vi "HMI.vi"(8 "error in (no error)":errorcluster caption="entrée d'erreur (pas d'erreur)", 11 "Class Popup WaitDIO en entrée":refnum<class "Class Popup WaitDIO.lvclass">) -> (0 "error out":errorcluster caption="sortie d'erreur", 1 "Input":string, 2 "Operator_Selection":bool, 3 "Class Popup WaitDIO en sortie":refnum<class "Class Popup WaitDIO.lvclass">)   [LabVIEW 2020, in "Library Instrument & Equipement.lvlib" / "Library Popup.lvlib" / "Class Popup WaitDIO.lvclass"]
uses:
  Class Popup WaitDIO.lvclass
  C:/Users/ngarcin/OneDrive - Altyor/Standard TB/Class/Popup/Class Popup (Main)/Class Popup (Main).lvclass
  C:/Users/ngarcin/OneDrive - Altyor/Standard TB/Class/Popup/Class Popup Operator_Validation/Class Popup Operator_Validation (Default)/Class Popup Operator_Validation (Virtual).lvclass
  Commun VI/TypeDef/Liste Error.ctl
  JSON API/JSON Value/Set from JSON string.vi
  Instrument/Instrument (Default)/Class Instrument (Default).lvclass
  JSON API/JSON Value/JSON Value.lvclass
  Class Popup Operator_Validation/Class Popup Operator_Validation (Default)/Class Popup Operator_Validation (Virtual).lvclass
  Class Popup WaitDIO.lvclass/Class Popup WaitDIO.ctl
  JSON API/Variant JSON/Variant JSON.lvlib
  JSON API/Get Polymorphic/JSON GetSet.lvlib
  Commun VI/Library Commun.lvlib
panel:
  out "Json_String":string
  out "Image":picture
  out "Text":string
  in  "Bouton NOK":bool caption="Default"
  in  "Bouton OK":bool caption="Validated"
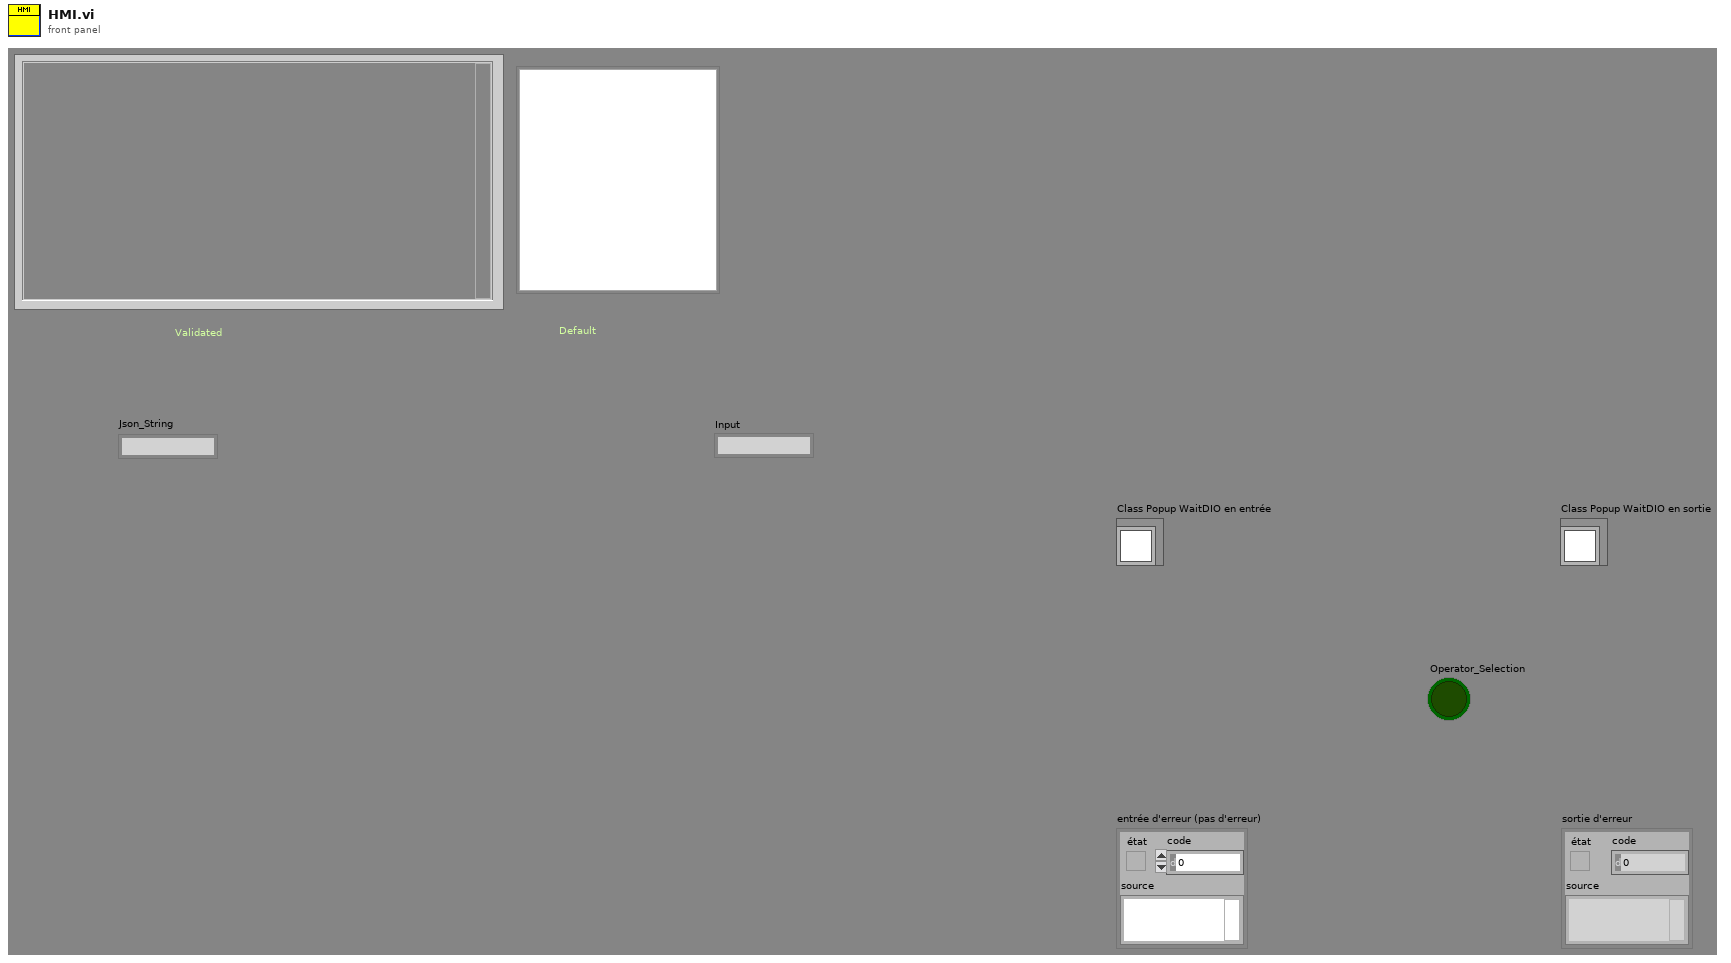
[diagram p1: front panel]
types:
  T1 = cluster{"Instrument":refnum<class "Class Instrument (Default).lvclass">, "Valur for test":bool, "Timeout (ms)":u64}
  T2 = typedef "Library Commun.lvlib/Liste Error.ctl" = enum16{"Firebase Driver - Get Document", "Firebase Driver - Get Document With Where", "Firebase Driver - Delete Document", "Firebase Driver - Set Document", "Firebase Driver - Update Document", "Firebase Altyor - Search Document Bench", "Firebase Altyor - Class Not in Firebase", "Spectrum_Analyser - Timeout", "Relay Board - Qty Relay", "DIO - Pb Funtion", "Power_Supply - Peripherical not find", "Mutimeter - Peripherical not find", "Instrument - Function Not Used", "Instrument - Instrument name not specified", "Instrument - Allready Initialised", "Instrument - TimeOut", "Instrument - the instrument must be Initialise before", "Instrument - Frame Not received", "Instrument - Frame Nok", "Test - Initialise the File_for_Save", "Test - Timeout", "Test - Cmd Error", "FGV - Variable ", "BDD FireBase - Define Class", "SN - Class Not Define"}
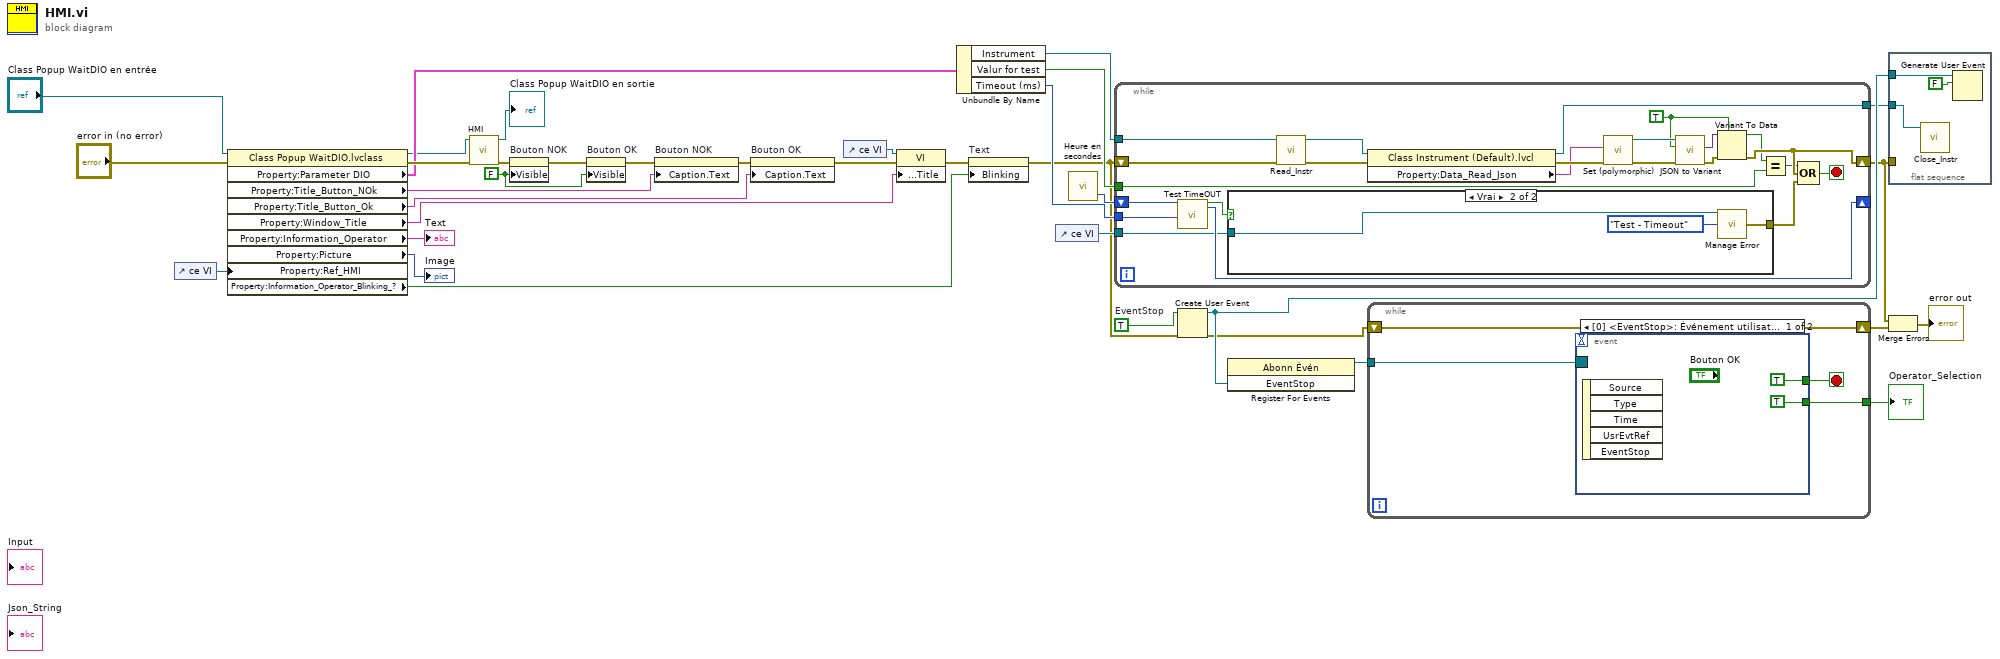
[diagram p0: block diagram]
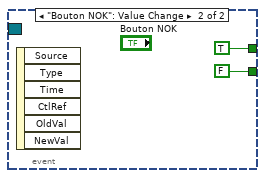
[diagram p3: hidden frame]
diagram:
  w18 = TRUE  # EventStop
  w22 = FALSE ("Visible")
  n1 = control-ref of="ce VI"() -> (w27:refnum<vi>)
  n2 = property class="Class Popup WaitDIO.lvclass"(reference="Class Popup WaitDIO en entrée", error in="error in (no error)", "Property:Ref_HMI"=w27) -> (reference out=w2:refnum<class "Class Popup WaitDIO.lvclass">, error out=w11:errorcluster, "Property:Parameter DIO"=w4:T1, "Property:Title_Button_NOk"=w35:string, "Property:Title_Button_Ok"=w36:string, "Property:Window_Title"=w30:string, "Property:Information_Operator"=→"Text":string, "Property:Picture"=→"Image":picture, "Property:Information_Operator_Blinking_?"=w25:bool)
  n3 = call-parent "HMI.vi"("error in (no error)"=w11, "Class Popup Operator_Validation (Default) en entrée"=w2) -> ("error out"=w3:errorcluster, "Class Popup Operator_Validation (Default) en sortie"=→"Class Popup WaitDIO en sortie":refnum<class "Class Popup WaitDIO.lvclass">)  [unwired: 6 in, 2 out]
  n4 = property on="Bouton NOK" class="Bool"(error in=w3, "Visible"=w22) -> (error out=w34:errorcluster)  [unwired: 1 in, 1 out]
  n5 = property on="Bouton OK" class="Bool"(error in=w34, "Visible"=w22) -> (error out=w33:errorcluster)  [unwired: 1 in, 1 out]
  n6 = property on="Bouton NOK" class="Bool"(error in=w33, "Caption.Text"=w35) -> (error out=w32:errorcluster)  [unwired: 1 in, 1 out]
  n7 = property on="Bouton OK" class="Bool"(error in=w32, "Caption.Text"=w36) -> (error out=w10:errorcluster)  [unwired: 1 in, 1 out]
  n8 = control-ref of="ce VI"() -> (w31:refnum<vi>)
  n9 = property class="VI"(reference=w31, error in=w10, "Front Panel.Title"=w30) -> (error out=w26:errorcluster)  [unwired: 1 out]
  n10 = Unbundle By Name(w4) -> ("Instrument"=w7:refnum<class "Class Instrument (Default).lvclass">, "Valur for test"=w12:bool, "Timeout (ms)"=w13:u64)
  n11 = property on="Text" class="Ch"(error in=w26, "Blinking"=w25) -> (error out=w6:errorcluster)  [unwired: 1 in, 1 out]
  n12 = control-ref of="ce VI"() -> (w20:refnum<vi>)
  n13 = call "Heure en secondes.vi"() -> ("Heure en milisecondes"=w21:u32)  [unwired: 2 in, 1 out]
  n14 = while {
    tunnel: w7 -> [w59]
    shift-right: [w48] -> w14
    shift-left: w6 -> [w58]
    tunnel: w13 -> [w44]
    shift-right: [w45] -> _
    shift-left: w21 -> [w46]
    tunnel: w20 -> [w43]
    tunnel: w12 -> [w39]
    tunnel: [w37] -> w8
    stop <- w47 stop-if-true
    w52 = TRUE
    n15 = call "Test TimeOUT.vi"("OLD Time"=w46, "TimeOut ms"=w44) -> ("Timeout ?"=w42:bool, "NEW Time"=w45:u32)  [unwired: 13 in, 3 out]
    n16 = case shown="Vrai" w42 {
      tunnel: w43 -> [_ w61]
      tunnel: [_ w60] -> w41
      frame False {
      }
      frame True {
        n17 = call "Manage Error.vi"("VI in Error"=w61, "Code Erreur"=Liste_Error."Test - Timeout") -> ("error out"=w60:errorcluster)  [unwired: 13 in]
      }
    }
    n18 = call-dynamic "Read_Instr.vi"("error in (no error)"=w58, "Class Instrument (Default) en entrée"=w59) -> ("error out"=w49:errorcluster, "Class Instrument (Default) en sortie"=w57:refnum<class "Class Instrument (Default).lvclass">)  [unwired: 8 in]
    n19 = property class="Class Instrument (Default).lvcl"(reference=w57, error in=w49) -> (reference out=w37:refnum<class "Class Instrument (Default).lvclass">, error out=w51:errorcluster, "Property:Data_Read_Json"=w50:string)
    n20 = call-poly "Set (polymorphic).vi"("error in (no error)"=w51, "JSON stream"=w50) -> ("error out"=w55:errorcluster, "JSON Value out"=w53:refnum<class "JSON Value.lvclass">)  [unwired: 7 in, 1 out]
    n21 = call "JSON to Variant.vi"("error in (no error)"=w55, "Variant (Data Type)"=w52, "JSON Value"=w53) -> ("error out"=w54:errorcluster, "Variant out"=w56:variant)  [unwired: 7 in]
    n22 = Variant To Data(error in=w54, type=w52, Variant=w56) -> (data=w40:bool, error out=w48:errorcluster)
    n23 = Equal?(x=w40, y=w39) -> (x = y?=w38:bool)
    n24 = Compound Arithmetic op=OR ("Opérateur arithmétique")(w38, w48, w41) -> (w47:bool)
  }
  n25 = Create User Event(user event datatype=w18, error in=w6) -> (user event=w17:refnum<user-event>, error out=w9:errorcluster)
  n26 = register-events(w17) -> (reference out=w19:refnum<event-registration>)  [unwired: 2 in, 1 out]
  n27 = while {
    tunnel: [w64] -> w23
    shift-right: [w65] -> w15
    shift-left: w9 -> [w65]
    tunnel: w19 -> [w63]
    stop <- w66 stop-if-true
    n28 = event shown="[0] <EventStop>: Événement utilisateur" {
      selector: w63 -> [_ _]
      dyn-events: _ -> [_ _]
      timeout: _ -> [_ _]
      tunnel: [TRUE ("Valeur (Signalisation)") TRUE ("Valeur (Signalisation)")] -> w66
      tunnel: [TRUE ("Operator_Selection") FALSE ("Operator_Selection")] -> w64
      event User Event {
        n29 = event-data() -> ()  [unwired: 1 in, 5 out]
      }
      event "Bouton NOK": Value Change {
        n30 = event-data() -> ()  [unwired: 1 in, 6 out]
      }
    }
  }
  "Operator_Selection" <- w23
  n31 = flat-sequence {
    tunnel: w17 -> [w73]
    tunnel: w14 -> [_]
    tunnel: w8 -> [w71]
    frame #0 {
      n32 = call-dynamic "Close_Instr.vi"("Class Instrument (Default) en entrée"=w71) -> ()  [unwired: 9 in, 2 out]
      n33 = Generate User Event(user event=w73, event data cluster=FALSE ("données d'événement")) -> ()  [unwired: 2 in, 2 out]
    }
  }
  n34 = Merge Errors(w14, w15) -> (→"error out":errorcluster)
